vi "PXI-4130 Init Channel (RT).vi"(5 "Channel Type":T3 items=["Voltage Controlled", "Current Controlled"], 7 "Channel Sense":T2=1008 items=["Local"=1008, "Remote"=1009], 8 "error in (no error)":errorcluster, 9 "Channel Name":string, 10 "resource name":refnum<k15>="Dev1", 11 "Device Reference In":T1 format="%.0x") -> (0 "error out":errorcluster, 2 "resource name Out":refnum<k15>="Dev1", 3 "Device Reference Out":T1 format="%.0x")   [LabVIEW 2009, in "PXI-4130 Custom Device.lvlib"]
uses:
  PXI-4130 Custom Device.lvlib
  Channel Type.ctl
  Channel Sense.ctl
  <vilib>/NI VeriStand/Custom Device API/Custom Device Item Ref.ctl
  <vilib>/NI VeriStand/Custom Device API/Custom Device Channel Type.ctl
  <instrlib>/niDCPower/nidcpower.llb/niDCPower Output Function.ctl
  <vilib>/NI VeriStand/Custom Device API/Custom Device API.lvlib
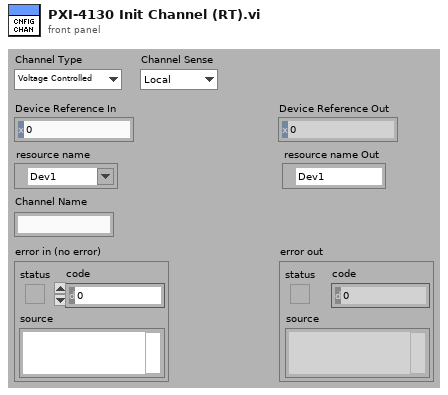
[diagram p1: front panel]
types:
  T1 = typedef "Custom Device API.lvlib/Custom Device Item Ref.ctl" = u64
  T2 = typedef "PXI-4130 Custom Device.lvlib/Channel Sense.ctl" = i32
  T3 = typedef "PXI-4130 Custom Device.lvlib/Channel Type.ctl" = i32
  T4 = typedef "Custom Device API.lvlib/Custom Device Channel Type.ctl" = enum16{"Input", "Output"}
  T5 = typedef "niDCPower Output Function.ctl" = i32
  T6 = typedef "Custom Device API.lvlib/Custom Device Channel.ctl" = cluster{"Type":T4, "Units":string, "Default Value":dbl, "Faultable":bool, "Scalable":bool}
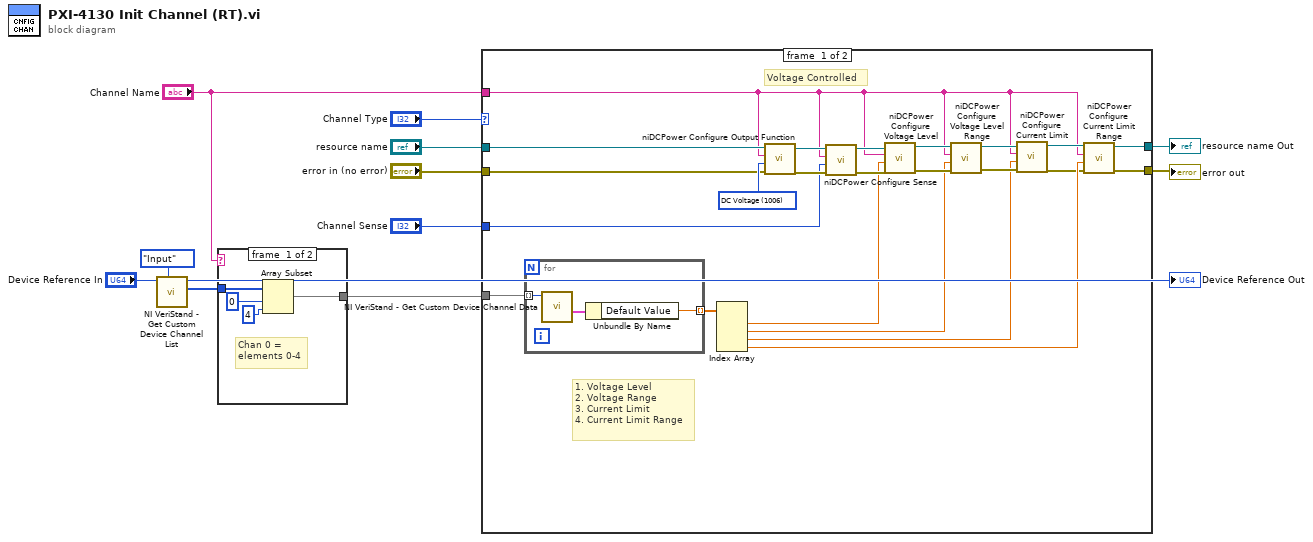
[diagram p0: block diagram]
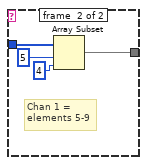
[diagram p2: hidden frame]
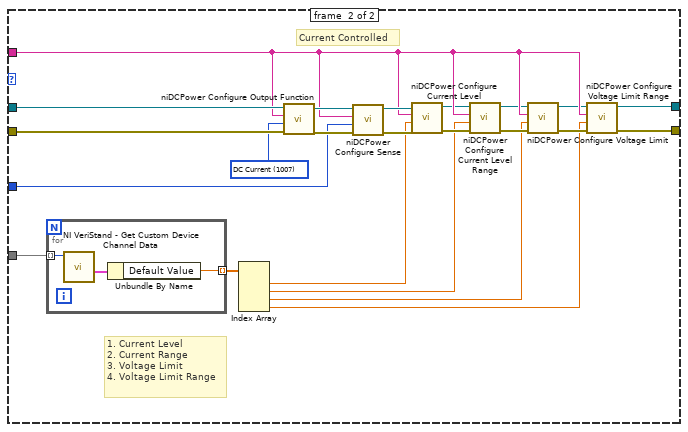
[diagram p3: hidden frame]
diagram:
  n1 = call <vilib>:"NI VeriStand - Get Custom Device Channel List.vi"("Channel Type"=Custom_Device_Channel_Type."Input", "Device Ref in"="Device Reference In") -> ("Specified Channel Ref List"=w5:T1[], "Device Ref out"=→"Device Reference Out":T1)  [unwired: 1 in, 7 out]
  n2 = case shown="\"1\"" "Channel Name" {
    tunnel: w5 -> [w16 w20]
    tunnel: [w13 w17] -> w4
    frame #0 {
      # "Chan 0 = \nelements 0-4"
      n3 = Array Subset(array=w16, index=0, length=4 ("index")) -> (w13:T1[])
    }
    frame #1 {
      # "Chan 1 = \nelements 5-9"
      n4 = Array Subset(array=w20, index=5, length=4 ("index")) -> (w17:T1[])
    }
  }
  n5 = case shown="1" "Channel Type" {
    tunnel: "error in (no error)" -> [w40 w62]
    tunnel: "resource name" -> [w39 w63]
    tunnel: "Channel Sense" -> [w36 w57]
    tunnel: [w35 w65] -> w1
    tunnel: [w34 w64] -> w2
    tunnel: "Channel Name" -> [w21 w60]
    tunnel: w4 -> [w32 w59]
    frame #0 {
      w43 = T5 1006 items=["DC Voltage"=1006, "DC Current"=1007] ("output function")
      # "1. Voltage Level\n2. Voltage Range\n3. Current Limit\n4. Current Limit Range"
      # "Voltage Controlled"
      n6 = for {
        tunnel: w32 -> [w45] mode=indexing
        tunnel: [w44] -> w33 mode=indexing
        n7 = call <vilib>:"NI VeriStand - Get Custom Device Channel Data.vi"("Channel Ref in"=w45) -> ("Channel"=w46:T6)  [unwired: 5 in, 5 out]
        n8 = Unbundle By Name(w46) -> ("Default Value"=w44:dbl)
      }
      n9 = Index Array(array=w33) -> (element #1=w31:dbl, element #2=w23:dbl, element #3=w22:dbl, element #4=w30:dbl)  [unwired: 4 in]
      n10 = call <instrlib>:"niDCPower Configure Output Function.vi"("error in (no error)"=w40, "output function"=w43, "channel name"=w21, "instrument handle"=w39) -> ("error out"=w41:errorcluster, "instrument handle out"=w42:refnum<k15>)  [unwired: 6 in]
      n11 = call <instrlib>:"niDCPower Configure Sense.vi"("error in (no error)"=w41, "sense"=w36, "channel name"=w21, "instrument handle"=w42) -> ("error out"=w38:errorcluster, "instrument handle out"=w37:refnum<k15>)  [unwired: 6 in]
      n12 = call <instrlib>:"niDCPower Configure Voltage Level.vi"("error in (no error)"=w38, "voltage level"=w31, "channel name"=w21, "instrument handle"=w37) -> ("error out"=w24:errorcluster, "instrument handle out"=w29:refnum<k15>)  [unwired: 6 in]
      n13 = call <instrlib>:"niDCPower Configure Voltage Level Range.vi"("error in (no error)"=w24, "voltage level range"=w23, "channel name"=w21, "instrument handle"=w29) -> ("error out"=w25:errorcluster, "instrument handle out"=w28:refnum<k15>)  [unwired: 6 in]
      n14 = call <instrlib>:"niDCPower Configure Current Limit.vi"("error in (no error)"=w25, "current limit"=w22, "channel name"=w21, "instrument handle"=w28) -> ("error out"=w26:errorcluster, "instrument handle out"=w27:refnum<k15>)  [unwired: 6 in]
      n15 = call <instrlib>:"niDCPower Configure Current Limit Range.vi"("error in (no error)"=w26, "current limit range"=w30, "channel name"=w21, "instrument handle"=w27) -> ("error out"=w34:errorcluster, "instrument handle out"=w35:refnum<k15>)  [unwired: 6 in]
    }
    frame #1 {
      w61 = T5 1007 items=["DC Voltage"=1006, "DC Current"=1007] ("output function")
      # "1. Current Level\n2. Current Range\n3. Voltage Limit\n4. Voltage Limit Range"
      # "Current Controlled"
      n16 = for {
        tunnel: w59 -> [w71] mode=indexing
        tunnel: [w70] -> w58 mode=indexing
        n17 = call <vilib>:"NI VeriStand - Get Custom Device Channel Data.vi"("Channel Ref in"=w71) -> ("Channel"=w72:T6)  [unwired: 5 in, 5 out]
        n18 = Unbundle By Name(w72) -> ("Default Value"=w70:dbl)
      }
      n19 = Index Array(array=w58) -> (element #1=w50:dbl, element #2=w49:dbl, element #3=w48:dbl, element #4=w47:dbl)  [unwired: 4 in]
      n20 = call <instrlib>:"niDCPower Configure Output Function.vi"("error in (no error)"=w62, "output function"=w61, "channel name"=w60, "instrument handle"=w63) -> ("error out"=w67:errorcluster, "instrument handle out"=w66:refnum<k15>)  [unwired: 6 in]
      n21 = call <instrlib>:"niDCPower Configure Sense.vi"("error in (no error)"=w67, "sense"=w57, "channel name"=w60, "instrument handle"=w66) -> ("error out"=w68:errorcluster, "instrument handle out"=w69:refnum<k15>)  [unwired: 6 in]
      n22 = call <instrlib>:"niDCPower Configure Current Level.vi"("error in (no error)"=w68, "current level"=w50, "channel name"=w60, "instrument handle"=w69) -> ("error out"=w51:errorcluster, "instrument handle out"=w52:refnum<k15>)  [unwired: 6 in]
      n23 = call <instrlib>:"niDCPower Configure Current Level Range.vi"("error in (no error)"=w51, "current level range"=w49, "channel name"=w60, "instrument handle"=w52) -> ("error out"=w53:errorcluster, "instrument handle out"=w56:refnum<k15>)  [unwired: 6 in]
      n24 = call <instrlib>:"niDCPower Configure Voltage Limit.vi"("error in (no error)"=w53, "voltage limit"=w48, "channel name"=w60, "instrument handle"=w56) -> ("error out"=w54:errorcluster, "instrument handle out"=w55:refnum<k15>)  [unwired: 6 in]
      n25 = call <instrlib>:"niDCPower Configure Voltage Limit Range.vi"("error in (no error)"=w54, "voltage limit range"=w47, "channel name"=w60, "instrument handle"=w55) -> ("error out"=w64:errorcluster, "instrument handle out"=w65:refnum<k15>)  [unwired: 6 in]
    }
  }
  "error out" <- w2
  "resource name Out" <- w1
